vi "11 Rings, Strings, and Tables.vi"() -> ()   [LabVIEW 2019]
uses:
  _Subs/OpenDiagram/Open_XControl.xctl
panel:
  in  "OpenDiag":refnum<vi>(xcontrol)
  out "where is the fox?":string
  out "Text output":string
  in  "Listbox":i32(listbox)=2
  out "Table Indicator":string[][](table)
  out "Output":string
  in  "Enum":enum16{"Tall", "Medium", "Short"}(ring)=enum."Medium"
  in  "Ring":u16(ring)=2 items=["One", "Two", "Three"]
  # "10 Rings, Strings, and Tables\nThis code shows different ways of using tables, strings, and rings\n\nInstructions:\n1. Hit the Run arrow and see what happens.\n2. Try selecting a different value in the ring, enum, or list box and run again.\n3. Check out the block diagram!"
  # "To edit ring / enum options, right click and go to Properties > Edit items..."
  # "Go to the block diagram for \nthis one!"
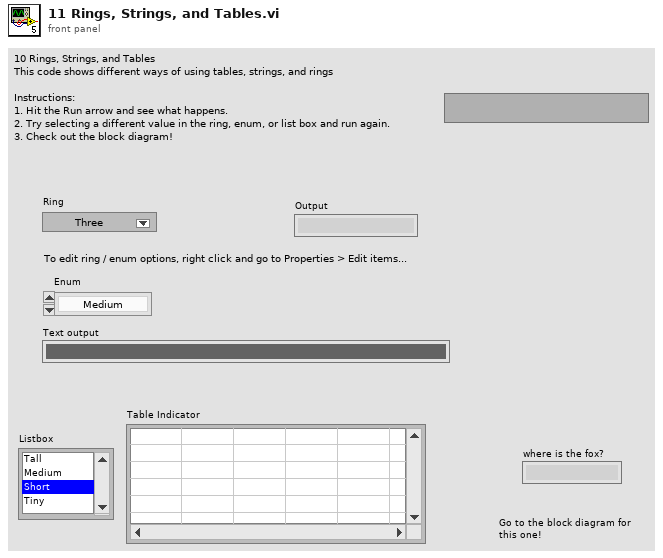
[diagram p1: front panel]
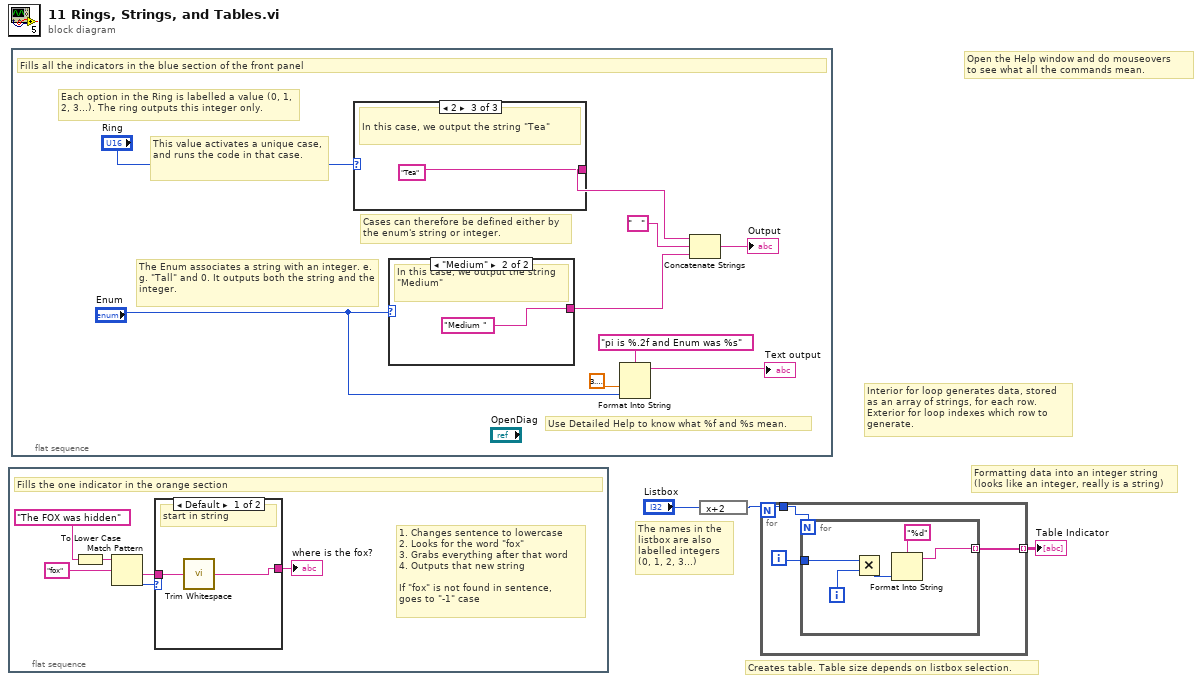
[diagram p0: block diagram]
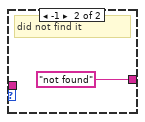
[diagram p2: hidden frame]
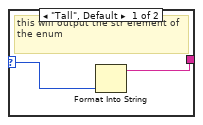
[diagram p3: hidden frame]
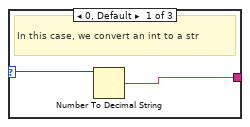
[diagram p4: hidden frame]
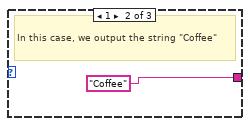
[diagram p5: hidden frame]
diagram:
  # "Interior for loop generates data, stored\nas an array of strings, for each row.\nExterior for loop indexes which row to \ngenerate."
  # "Creates table. Table size depends on listbox selection."
  # "Formatting data into an integer string\n(looks like an integer, really is a string)"
  # "The names in the \nlistbox are also \nlabelled integers \n(0, 1, 2, 3...)"
  # "Open the Help window and do mouseovers\nto see what all the commands mean."
  n1 = flat-sequence {
    frame #0 {
      # "1. Changes sentence to lowercase\n2. Looks for the word \"fox\"\n3. Grabs everything after that word\n4. Outputs that new string\n\nIf \"fox\" is not found in sentence, \ngoes to \"-1\" case"
      # "Fills the one indicator in the orange section"
      n2 = To Lower Case(string="The FOX was hidden" ("format string")) -> (all lower case string=w7:string)
      n3 = Match Pattern(string=w7, regular expression="fox") -> (after substring=w4:string, offset past match=w6:i32)  [unwired: 1 in, 2 out]
      n4 = case shown="Default" w6 {
        tunnel: [w10 "not found" ("regular expression")] -> w5
        tunnel: w4 -> [w11 _]
        frame Default {
          # "start in string"
          n5 = call <vilib>:"Trim Whitespace.vi"("string"=w11) -> ("trimmed string"=w10:string)  [unwired: 1 in]
        }
        frame -1 {
          # "did not find it"
        }
      }
      "where is the fox?" <- w5
    }
  }
  n6 = flat-sequence {
    frame #0 {
      # "Use Detailed Help to know what %f and %s mean."
      # "Cases can therefore be defined either by the enum's string or integer."
      # "The Enum associates a string with an integer. e.g. \"Tall\" and 0. It outputs both the string and the integer."
      # "This value activates a unique case, and runs the code in that case."
      # "Each option in the Ring is labelled a value (0, 1, 2, 3...). The ring outputs this integer only."
      # "Fills all the indicators in the blue section of the front panel"
      n7 = case shown="2" "Ring" {
        selector: "Ring" -> [w26 _ _]
        tunnel: [w25 "Coffee" "Tea"] -> w19
        frame 0, Default {
          # "In this case, we convert an int to a str"
          n8 = Number To Decimal String(number=w26) -> (decimal integer string=w25:string)  [unwired: 1 in]
        }
        frame 1 {
          # "In this case, we output the string \"Coffee\""
        }
        frame 2 {
          # "In this case, we output the string \"Tea\""
        }
      }
      n9 = case shown="\"Medium\"" "Enum" {
        selector: "Enum" -> [w23 _]
        tunnel: [w22 "Medium "] -> w20
        frame "Tall", Default {
          # "this will output the str element of the enum"
          n10 = Format Into String(w23) -> (resulting string=w22:string)  [unwired: 3 in, 1 out]
        }
        frame "Medium" {
          # "In this case, we output the string  \"Medium\""
        }
      }
      n11 = Format Into String(format string="pi is %.2f and Enum was %s", 3.141592653589793, "Enum") -> (resulting string=→"Text output":string)  [unwired: 2 in, 1 out]
      n12 = Concatenate Strings(w19, "   " ("string"), w20) -> (→"Output":string)
    }
  }
  n13 = expression code="x+2"("Listbox") -> (w2:i32)
  n14 = for {
    N: w2 -> [_]
    tunnel: w2 -> [w31]
    tunnel: [w30] -> w3 mode=indexing
    i -> [w29]
    n15 = for {
      N: w31 -> [_]
      tunnel: [w35] -> w30 mode=indexing
      tunnel: w29 -> [w34]
      i -> [w33]
      n16 = Multiply(x=w34, y=w33) -> (x*y=w32:i32)
      n17 = Format Into String(format string="%d", w32) -> (resulting string=w35:string)  [unwired: 2 in, 1 out]
    }
  }
  "Table Indicator" <- w3
